vi "Write_attrib_array.vi"(4 "attribs":variant[](array[variant]), 5 "prefix":string, 6 "error in (no error)":errorcluster, 7 "overwrite?":bool, 8 "obj_name":string=".", 9 "ref":i32) -> (0 "error out":errorcluster, 3 "ref out":i32)   [LabVIEW 2010]
doc: "Writes a 1D-array of variants to the given object/id. The name of each attribute written is the name associated with the variant, with the specified prefix attached."
uses:
  <vilib>/Utility/VariantDataType/VariantType.lvlib
  <vilib>/addons/h5labview2/attrib/H5A.lvlib
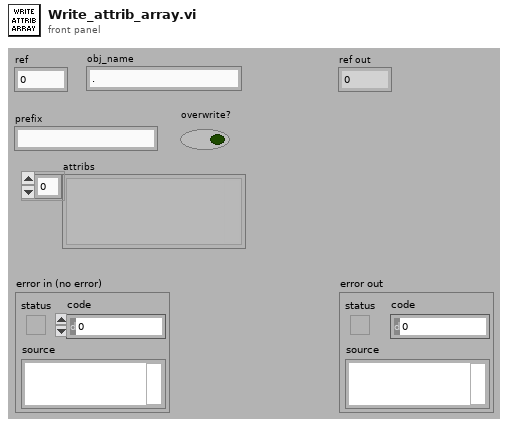
[diagram p1: front panel]
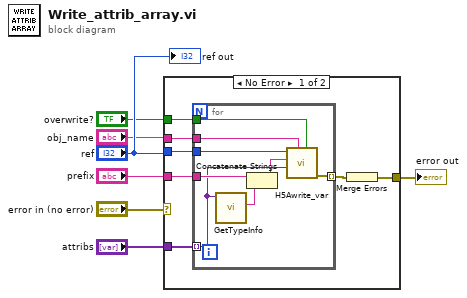
[diagram p0: block diagram]
diagram:
  n1 = case shown="No Error" "error in (no error)" {
    selector: "error in (no error)" -> [_ w23]
    tunnel: [w13 w23] -> w5
    tunnel: "prefix" -> [w12 _]
    tunnel: "attribs" -> [w11 _]
    tunnel: "ref" -> [w10 _]
    tunnel: "overwrite?" -> [w9 _]
    tunnel: "obj_name" -> [w8 _]
    frame No Error {
      n2 = for {
        tunnel: w9 -> [w17]
        tunnel: [w22] -> w14 mode=indexing
        tunnel: w12 -> [w21]
        tunnel: w11 -> [w19] mode=indexing
        tunnel: w10 -> [w18]
        tunnel: w8 -> [w16]
        n3 = call <vilib>:"GetTypeInfo.vi"("Variant"=w19) -> ("Name"=w20:string)  [unwired: 6 in, 4 out]
        n4 = Concatenate Strings(w21, w20) -> (w15:string)
        n5 = call <vilib>:"H5Awrite_var.vi"("replace? (T)"=w17, "object name"=w16, "data"=w19, "attrib name"=w15, "ref in"=w18) -> ("error out"=w22:errorcluster)  [unwired: 3 in, 2 out]
      }
      n6 = Merge Errors(w14) -> (w13:errorcluster)
    }
    frame Error {
    }
  }
  "error out" <- w5
  "ref out" <- "ref"
